vi "UserConsoleFGV.vi"(8 "error in (no error)":errorcluster, 10 "Deposit Amount In":dbl, 11 "Enum":T1(ring)) -> (0 "error out":errorcluster, 2 "Deposit Amount out":dbl)   [LabVIEW 2013, in "UserConsole.lvlib"]
uses:
  UserConsole.lvlib
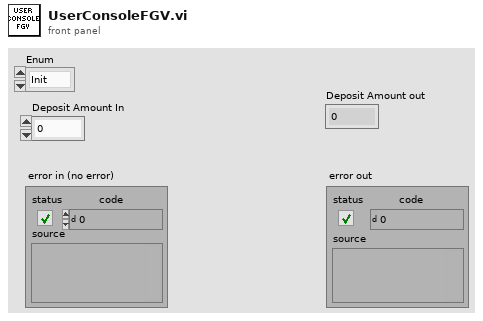
[diagram p1: front panel]
types:
  T1 = enum16{"Init", "Set Variables", "Get Variables", "Clear"}
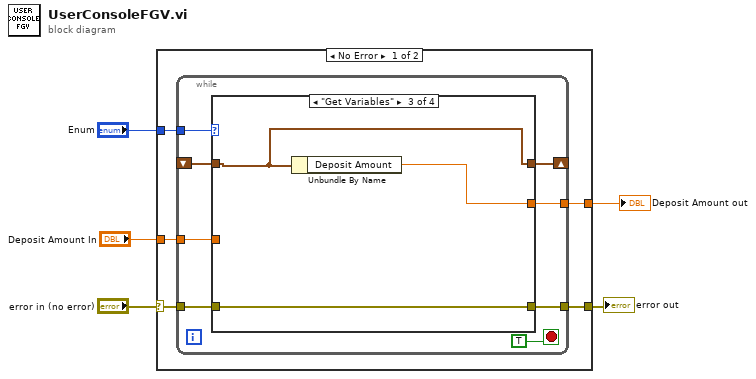
[diagram p0: block diagram]
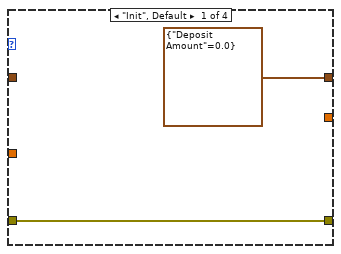
[diagram p2: hidden frame]
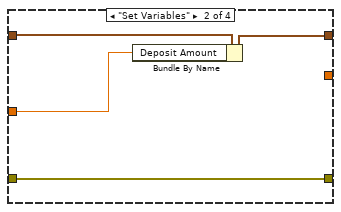
[diagram p3: hidden frame]
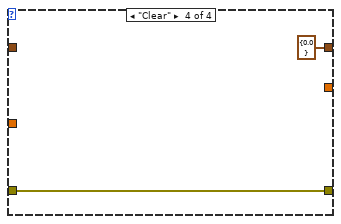
[diagram p4: hidden frame]
diagram:
  n1 = case shown="No Error" "error in (no error)" {
    selector: "error in (no error)" -> [w10 w30]
    tunnel: [w9 w30] -> w4
    tunnel: "Enum" -> [w8 _]
    tunnel: "Deposit Amount In" -> [w7 _]
    tunnel: [w6 _] -> w1
    frame No Error {
      n2 = while {
        tunnel: w10 -> [w17]
        tunnel: [w16] -> w9
        tunnel: w8 -> [w18]
        shift-right: [w15] -> _
        shift-left: _ -> [w14]
        tunnel: w7 -> [w13]
        tunnel: [w12] -> w6
        stop <- TRUE stop-if-true
        n3 = case shown="\"Get Variables\"" w18 {
          tunnel: w17 -> [w20 w24 w27 w29]
          tunnel: [w20 w24 w27 w29] -> w16
          tunnel: [cluster{"Deposit Amount":dbl} {"Deposit Amount"=0.0} w22 w25 cluster{"Deposit Amount":dbl} {"Deposit Amount"=0.0}] -> w15
          tunnel: w14 -> [_ w23 w25 _]
          tunnel: w13 -> [_ w21 _ _]
          tunnel: [_ _ w26 _] -> w12
          frame "Init", Default {
          }
          frame "Set Variables" {
            n4 = Bundle By Name(cluster=w23, "Deposit Amount"=w21) -> (w22:cluster{"Deposit Amount":dbl})
          }
          frame "Get Variables" {
            n5 = Unbundle By Name(w25) -> ("Deposit Amount"=w26:dbl)
          }
          frame "Clear" {
          }
        }
      }
    }
    frame Error {
    }
  }
  "error out" <- w4
  "Deposit Amount out" <- w1
